vi "圖片辨識.vi"() -> ()   [LabVIEW 2021]
uses:
  <vilib>/vision/NI_Vision_Development_Module.lvlib
panel:
  out "Segmented Image":T1(plugin-control)
  in  "Number of Classes":i32=2
  out "Threshold Data out":T2(array[cluster]) {"Replace Value" format="%.2f"; "Upper value" format="%.2f"; "Lower value" format="%.2f"}
  out "Threshold Image":T1(plugin-control)
  out "Labeled Image":T1(plugin-control)
  out "Before Threshold":T1(plugin-control)
  in  "Connectivity 4/8 (8)":bool=TRUE
  in  "Range":cluster{"Lower value":sgl, "Upper value":sgl}={"Lower value"=128.0, "Upper value"=255.0} {"Upper value" scale=0.0..255.0; "Lower value" scale=0.0..255.0}
  in  "stop":bool
  in  "File Path":path
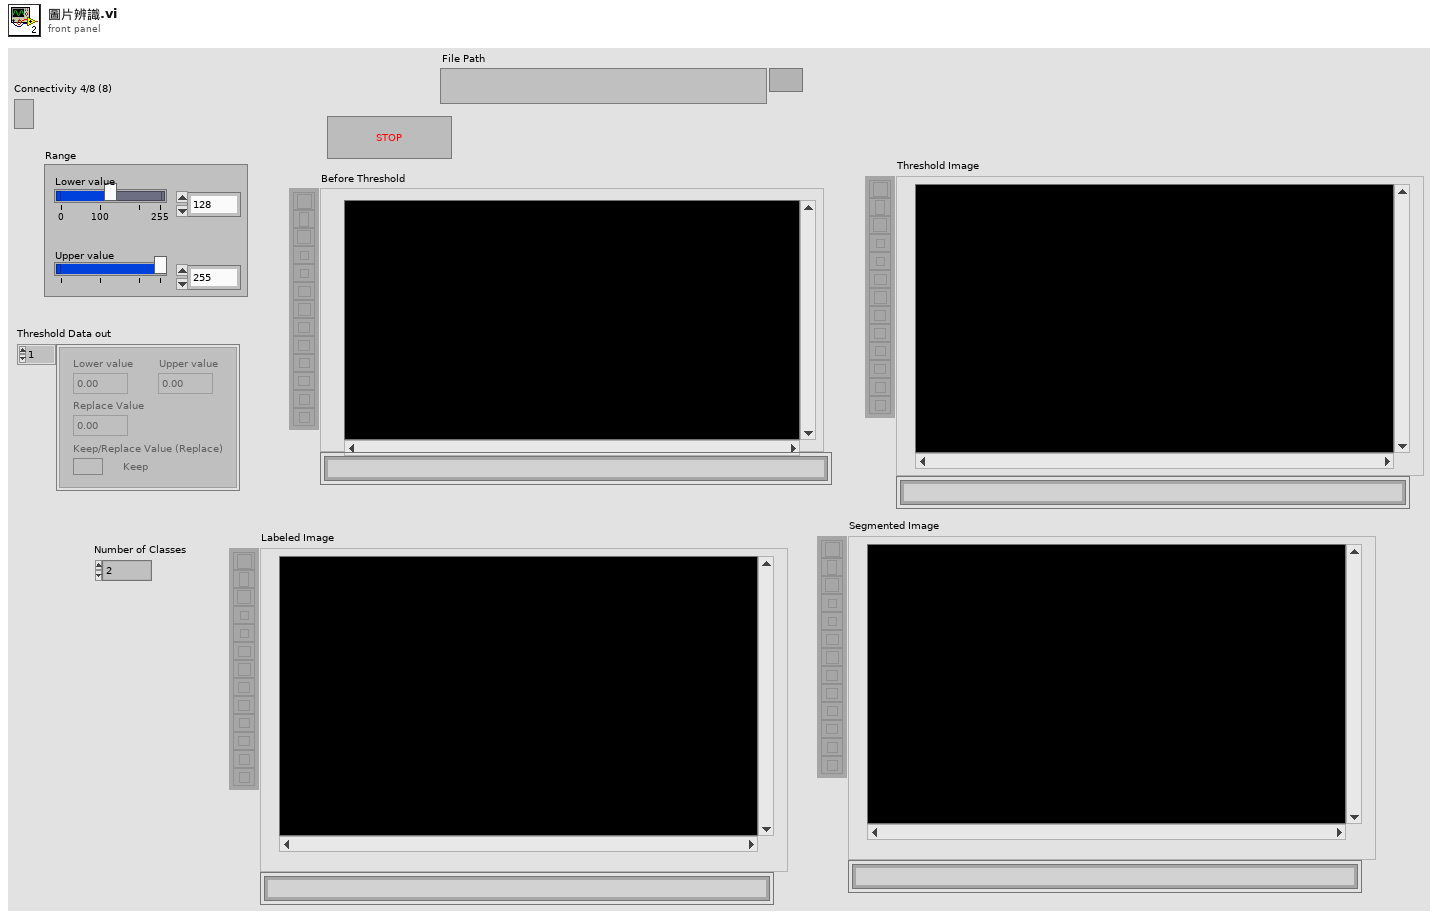
[diagram p1: front panel]
types:
  T1 = typedef "IMAQ Image.ctl" = refnum<image>
  T2 = cluster{"Lower value":sgl, "Upper value":sgl, "Replace Value":sgl, "Keep/Replace Value (Replace)":bool}[]
  T3 = enum32{"AutoM", "Close", "Dilate", "Erode", "Gradient", "Gradient out", "Gradient in", "Hit miss", "Open", "PClose", "POpen", "Thick", "Thin"}
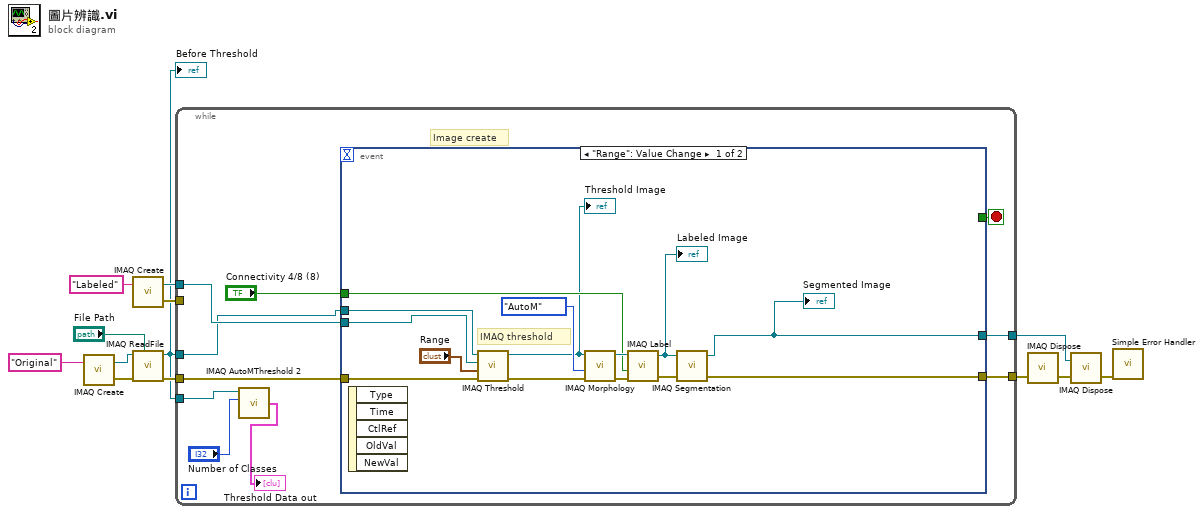
[diagram p0: block diagram]
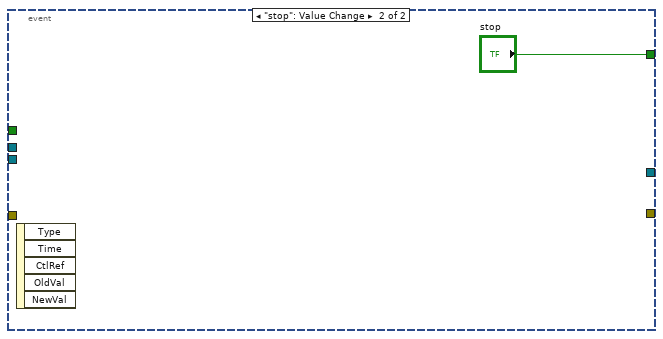
[diagram p2: hidden frame]
diagram:
  n1 = call "IMAQ Create"("Image Name"="Original") -> ("New Image"=w13:T1, "error out"=w7:errorcluster)  [unwired: 4 in]
  n2 = call "IMAQ Create"("Image Name"="Labeled") -> ("New Image"=w11:T1, "error out"=w10:errorcluster)  [unwired: 4 in]
  n3 = call "IMAQ ReadFile"("File Path"="File Path", "error in (no error)"=w7, "Image"=w13) -> ("error out"=w6:errorcluster, "Image Out"=w1:T1)  [unwired: 4 in, 3 out]
  "Before Threshold" <- w1
  n4 = while {
    tunnel: w1 -> [w22]
    tunnel: w11 -> [w23]
    tunnel: w10 -> [_]
    tunnel: w6 -> [w19]
    tunnel: [w18] -> w3
    tunnel: [w17] -> w2
    tunnel: w1 -> [w16]
    stop <- w20 stop-if-true
    # "Image create"
    n5 = call "IMAQ AutoMThreshold 2"("Number of Classes"="Number of Classes", "Image"=w16) -> ("Threshold Data out"=→"Threshold Data out":T2)  [unwired: 2 in, 2 out]
    n6 = event shown="[0] \"Range\": Value Change" {
      selector: _ -> [_ _]
      dyn-events: _ -> [_ _]
      timeout: _ -> [_ _]
      tunnel: w23 -> [w26 _]
      tunnel: w19 -> [w29 _]
      tunnel: w22 -> [w28 _]
      tunnel: "Connectivity 4/8 (8)" -> [w34 _]
      tunnel: [_ "stop"] -> w20
      tunnel: [w30 _] -> w18
      tunnel: [w25 _] -> w17
      event "Range": Value Change {
        # "IMAQ threshold"
        n7 = event-data() -> ()  [unwired: 1 in, 5 out]
        n8 = call "IMAQ Threshold"("error in (no error)"=w29, "Range"="Range", "Image Dst"=w26, "Image Src"=w28) -> ("error out"=w33:errorcluster, "Image Dst Out"=w27:T1)  [unwired: 6 in]
        "Threshold Image" <- w27
        n9 = call "IMAQ Morphology"("error in (no error)"=w33, "Operation"=T3."AutoM", "Image Src"=w27) -> ("error out"=w32:errorcluster, "Image Dst Out"=w36:T1)  [unwired: 4 in, 3 out]
        n10 = call "IMAQ Label"("error in (no error)"=w32, "Connectivity 4/8 (8)"=w34, "Image Src"=w36) -> ("error out"=w31:errorcluster, "Image Dst Out"=w24:T1)  [unwired: 1 in, 1 out]
        "Labeled Image" <- w24
        n11 = call "IMAQ Segmentation"("error in (no error)"=w31, "Image Src"=w24) -> ("error out"=w30:errorcluster, "Image Dst Out"=w25:T1)  [unwired: 2 in]
        "Segmented Image" <- w25
      }
      event "stop": Value Change {
        n12 = event-data() -> ()  [unwired: 1 in, 5 out]
      }
    }
  }
  n13 = call "IMAQ Dispose"("error in (no error)"=w3) -> ("error out"=w5:errorcluster)  [unwired: 2 in, 3 out]
  n14 = call "IMAQ Dispose"("Image"=w2, "error in (no error)"=w5) -> ("error out"=w4:errorcluster)  [unwired: 1 in, 3 out]
  n15 = call <vilib>:"Simple Error Handler.vi"("error in (no error)"=w4) -> ()  [unwired: 1 in, 8 out]
